vi "Check_Loop_Error_FGV.vi"(8 "error in (no error)":errorcluster, 9 "queue IN":refnum<queue>, 10 "Ignore Errors":i32[](array[numeric]), 11 "Exit on Error? (F)":bool) -> (3 "Boolean":bool)   [LabVIEW 2024, in "PCANusb_DTU.lvlib"]
doc: "ThisVI\n---------------------------------------------------\nCheck Loop Error List\n---------------------------------------------------\n-Checks the Error Code .\n-Eneque the \"Exit\" or \"Error\" message if error code in Ignore Error List."
uses:
  PCANusb_DTU.lvlib
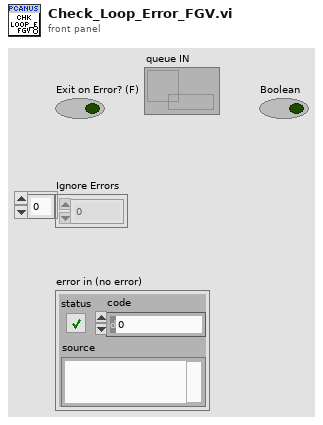
[diagram p1: front panel]
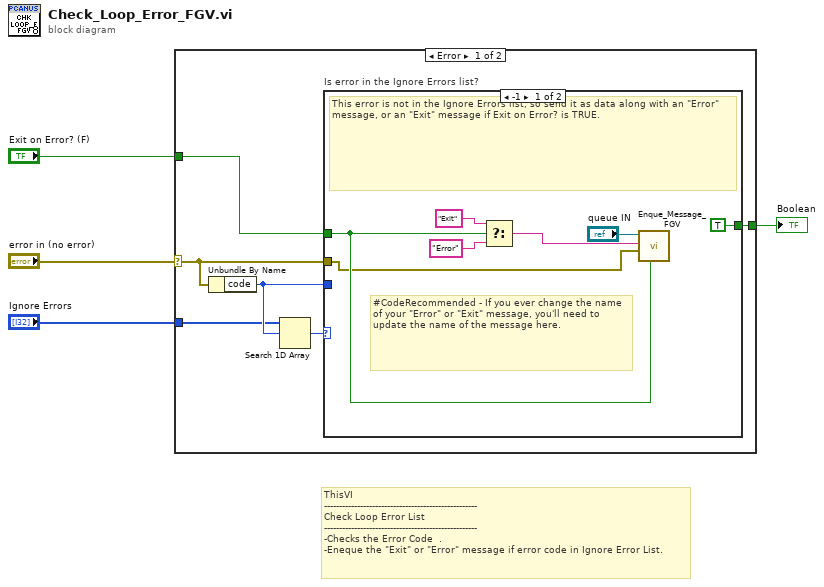
[diagram p0: block diagram]
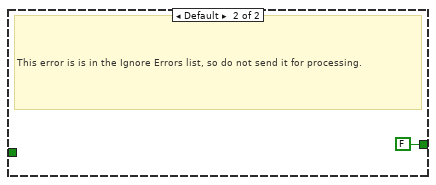
[diagram p2: hidden frame]
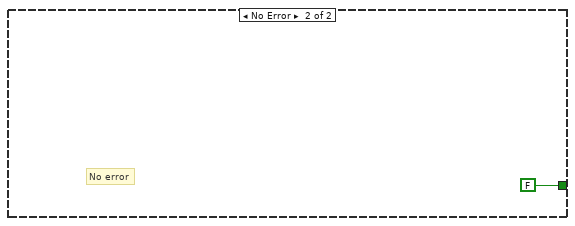
[diagram p3: hidden frame]
diagram:
  # "ThisVI\n---------------------------------------------------\nCheck Loop Error List\n---------------------------------------------------\n-Checks the Error Code  .\n-Eneque the \"Exit\" or \"Error\" message if error code in Ignore Error List."
  n1 = case shown="Error" "error in (no error)" {
    selector: "error in (no error)" -> [w8 _]
    tunnel: "Ignore Errors" -> [w7 _]
    tunnel: [w6 FALSE] -> w3
    tunnel: "Exit on Error? (F)" -> [w5 _]
    frame Error {
      n2 = Unbundle By Name(w8) -> ("code"=w9:i32)
      n3 = Search 1D Array(1D array=w7, element=w9) -> (index of element=w10:i32)  [unwired: 1 in]
      n4 = case "Is error in the Ignore Errors list?" shown="-1" w10 {
        tunnel: w8 -> [w13 _]
        tunnel: w9 -> [_ _]
        tunnel: [TRUE FALSE] -> w6
        tunnel: w5 -> [w14 _]
        frame -1 {
          # "#CodeRecommended - If you ever change the name of your \"Error\" or \"Exit\" message, you'll need to update the name of the message here."
          # "This error is not in the Ignore Errors list, so send it as data along with an \"Error\" message, or an \"Exit\" message if Exit on Error? is TRUE."
          n5 = Select(t="Exit" ("Message"), s=w14, f="Error" ("Message")) -> (s? t:f=w12:string)
          n6 = call "Enque_Message_FGV.vi"("Priority"=w14, "Message Data"=w13, "Message"=w12, "queue IN"="queue IN") -> ()  [unwired: 7 in, 1 out]
        }
        frame Default {
          # "This error is is in the Ignore Errors list, so do not send it for processing."
        }
      }
    }
    frame No Error {
      # "No error"
    }
  }
  "Boolean" <- w3
